vi "cost.vi"(8 "error in (no error)":errorcluster, 11 "Mocha in":refnum<class "Mocha.lvclass">) -> (0 "error out":errorcluster, 2 "Cost":dbl, 3 "Mocha out":refnum<class "Mocha.lvclass">)   [LabVIEW 2021, in "Mocha.lvclass"]
uses:
  Mocha.lvclass
  Beverage/Beverage.lvclass
panel:
  # "Connector Pane"
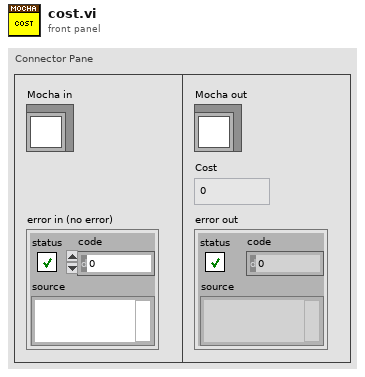
[diagram p1: front panel]
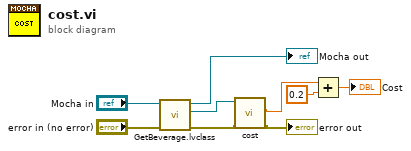
[diagram p0: block diagram]
diagram:
  n1 = call-dynamic "GetBeverage.lvclass.vi"("error in (no error)"="error in (no error)", "object in"="Mocha in") -> ("error out"=w3:errorcluster, "Beverage.lvclass"=w4:refnum<class "Beverage.lvclass">, "object out"=→"Mocha out":refnum<class "Mocha.lvclass">)  [unwired: 7 in]
  n2 = call-dynamic "cost.vi"("error in (no error)"=w3, "Beverage in"=w4) -> ("error out"=→"error out":errorcluster, "Cost"=w1:dbl)  [unwired: 7 in, 1 out]
  n3 = Add(x=w1, y=0.2) -> (x+y=→"Cost":dbl)
